vi "New Connection Handler.vi"(6 "Connection Handler in":refnum<class "Connection Handler.lvclass">, 7 "ID":i32, 8 "error in (no error)":errorcluster, 11 "Socket":refnum<class "Socket.lvclass">) -> (0 "error out":errorcluster, 3 "Connection Handler out":refnum<class "Connection Handler.lvclass">)   [LabVIEW 2017, in "Connection Handler.lvlib" / "Connection Handler.lvclass"]
uses:
  Connection Handler.lvclass
  <vilib>/MediaMongrels Ltd/WebSockets/Sockets/Socket/Socket.lvclass
  Connection Handler.lvclass/Connection Handler.ctl
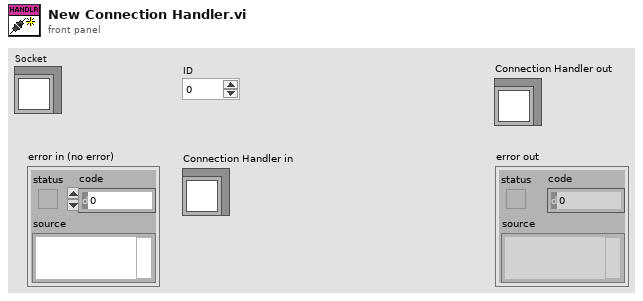
[diagram p1: front panel]
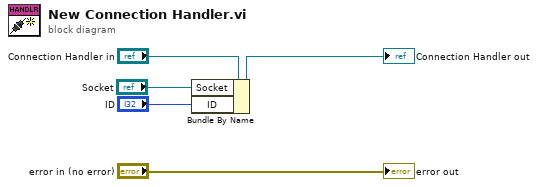
[diagram p0: block diagram]
diagram:
  n1 = Bundle By Name(cluster="Connection Handler in", "Socket"="Socket", "ID"="ID") -> (→"Connection Handler out":refnum<class "Connection Handler.lvclass">)
  "error out" <- "error in (no error)"
